vi "Read Desired Temperature.vi"(11 "Cooler in":refnum<class "Cooler.lvclass">) -> (2 "Desired Temperature":dbl=75.0)   [LabVIEW 2025, in "Cooler.lvlib" / "Cooler.lvclass"]
doc: "Reads the temperature that the system is aiming to maintain."
uses:
  Cooler.lvclass
  Level Controller/Level Controller/Level Controller.lvclass
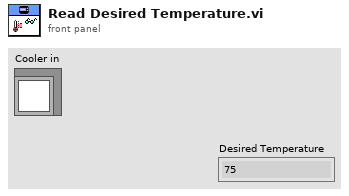
[diagram p1: front panel]
types:
  T1 = typedef "Level Controller.lvlib/Level Controller.lvclass/Deadband.ctl" = cluster{"Low":dbl, "High":dbl}
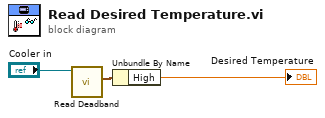
[diagram p0: block diagram]
diagram:
  n1 = call "Read Deadband.vi"("Level Controller in"="Cooler in") -> ("Deadband"=w2:T1)  [unwired: 8 in, 2 out]
  n2 = Unbundle By Name(w2) -> ("High"=→"Desired Temperature":dbl)
